vi "DSO1072B_BasicCMD.vi"(1 "AutoRead":bool, 4 "Delay(mS)":u32, 5 "byte count":u32, 6 "Read?":bool, 7 "ManualCMD?":bool, 8 "error in (no error)":errorcluster, 9 "DSO1072B CMD":string(combo), 10 "write buffer":string, 11 "VISA resource name In":refnum<visa-resource-name>) -> (0 "error out":errorcluster, 2 "read buffer":string, 3 "VISA resource name Out":refnum<visa-resource-name>)   [LabVIEW 2011]
panel:
  out "length":i32
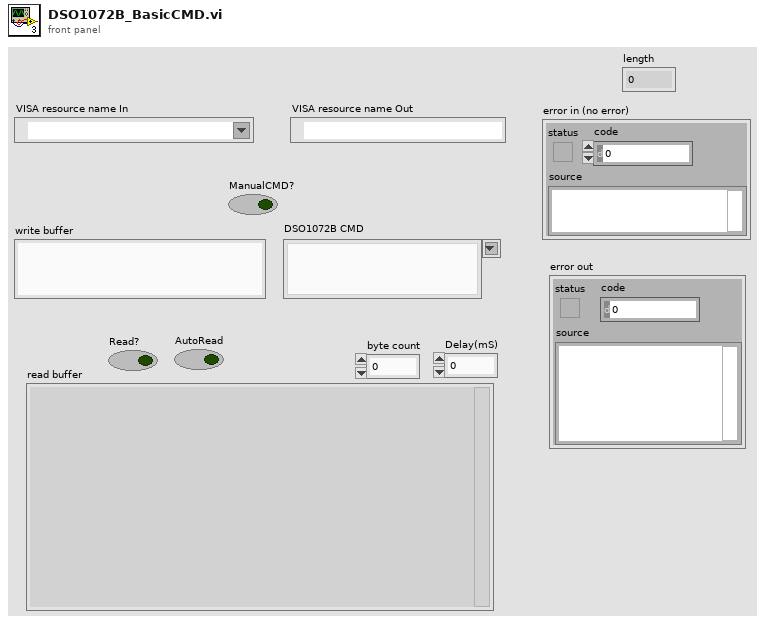
[diagram p1: front panel]
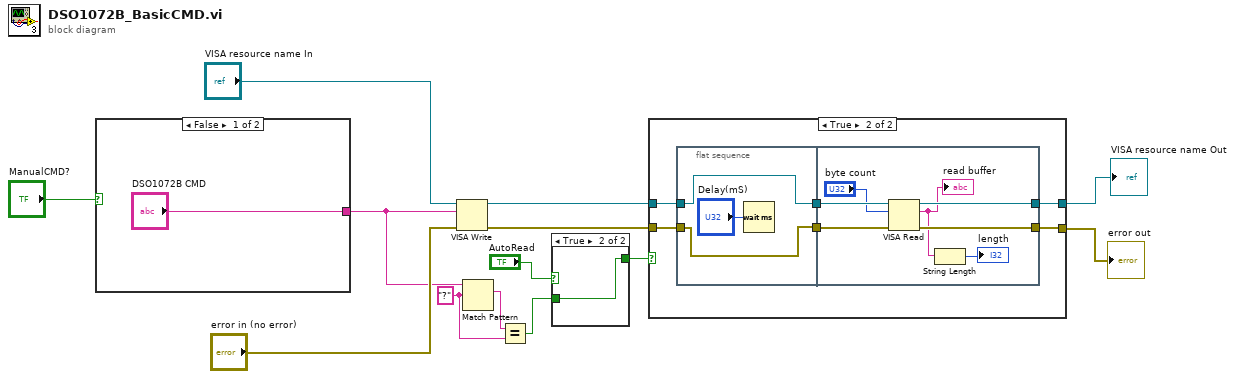
[diagram p0: block diagram]
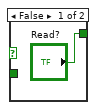
[diagram p2: hidden frame]
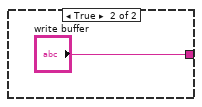
[diagram p3: hidden frame]
diagram:
  w3 = "?" ("regular expression")
  n1 = case shown="False" "ManualCMD?" {
    tunnel: ["DSO1072B CMD" "write buffer"] -> w5
    frame False {
    }
    frame True {
    }
  }
  n2 = VISA Write(VISA resource name="VISA resource name In", write buffer=w5, error in (no error)="error in (no error)") -> (VISA resource name out=w10:refnum<visa-resource-name>, error out=w9:errorcluster)  [unwired: 1 out]
  n3 = Match Pattern(string=w5, regular expression=w3) -> (match substring=w4:string)  [unwired: 1 in, 3 out]
  n4 = Equal?(x=w4, y=w3) -> (x = y?=w2:bool)
  n5 = case shown="True" "AutoRead" {
    tunnel: ["Read?" w17] -> w11
    tunnel: w2 -> [_ w17]
    frame False {
    }
    frame True {
    }
  }
  n6 = case shown="True" w11 {
    tunnel: w10 -> [w19 w25]
    tunnel: w9 -> [w18 w23]
    tunnel: [w19 w21] -> w7
    tunnel: [w18 w20] -> w8
    frame False {
    }
    frame True {
      n7 = flat-sequence {
        tunnel: w25 -> [w27]
        tunnel: [w27] -> w24
        tunnel: w23 -> [w26]
        tunnel: [w26] -> w22
        tunnel: w24 -> [w35]
        tunnel: w22 -> [w34]
        tunnel: [w32] -> w21
        tunnel: [w31] -> w20
        frame #0 {
          n8 = Wait (ms)(milliseconds to wait="Delay(mS)") -> ()  [unwired: 1 out]
        }
        frame #1 {
          n9 = VISA Read(VISA resource name=w35, byte count="byte count", error in (no error)=w34) -> (VISA resource name out=w32:refnum<visa-resource-name>, read buffer=w29:string, error out=w31:errorcluster)  [unwired: 1 out]
          "read buffer" <- w29
          n10 = String Length(string=w29) -> (length=→"length":i32)
        }
      }
    }
  }
  "error out" <- w8
  "VISA resource name Out" <- w7
